vi "GraphViz Generator UI Wrapper.vi"(10 "Modules Configurations":refnum<class "TBM module configuration.lvclass">[](array[class]), 11 "engine configuration in":refnum<class "engine configuration.lvclass">) -> ()   [LabVIEW 2013, in "GraphViz Mapping Visualizer.lvlib"]
uses:
  GraphViz Mapping Visualizer.lvlib
  <vilib>/NI/Module Execution Interface/Engine Configuration/engine configuration.lvclass
  <vilib>/NI/Tag Bus Module Framework/module configuration/TBM module configuration.lvclass
  System.Windows.Forms
  <vilib>/event_ctls.llb/panelstate.ctl
  <vilib>/event_ctls.llb/sizeaction.ctl
  System.Drawing
  Configuration Editor/Classes/Engine Mappings/Engine Mappings.lvclass
panel:
  in  "Tab Control":enum32{"Setup", "Image"}(tab)
  in  "Modules to View":T1(array[cluster])
  in  "Supported Colors":string[](array[string])=["dodgerblue", "cadetblue1", "darkgoldenrod1", "gainsboro", "palegreen", "peachpuff", "violet", "skyblue", "yellow", "seagreen1", "tomato", "thistle", "slateblue1", "orange", "palevioletred1"]
  in  "Show Unmapped Channels?":bool=TRUE
  in  "Show Tag Labels?":bool
  in  "Zoom?":bool=TRUE
  in  "Generate":bool
  in  "PictureBox":refnum<k24>(container)
  # "Generation Options"
  # "Supported colors list found at \nhttp://www.graphviz.org/doc/info/colors.html"
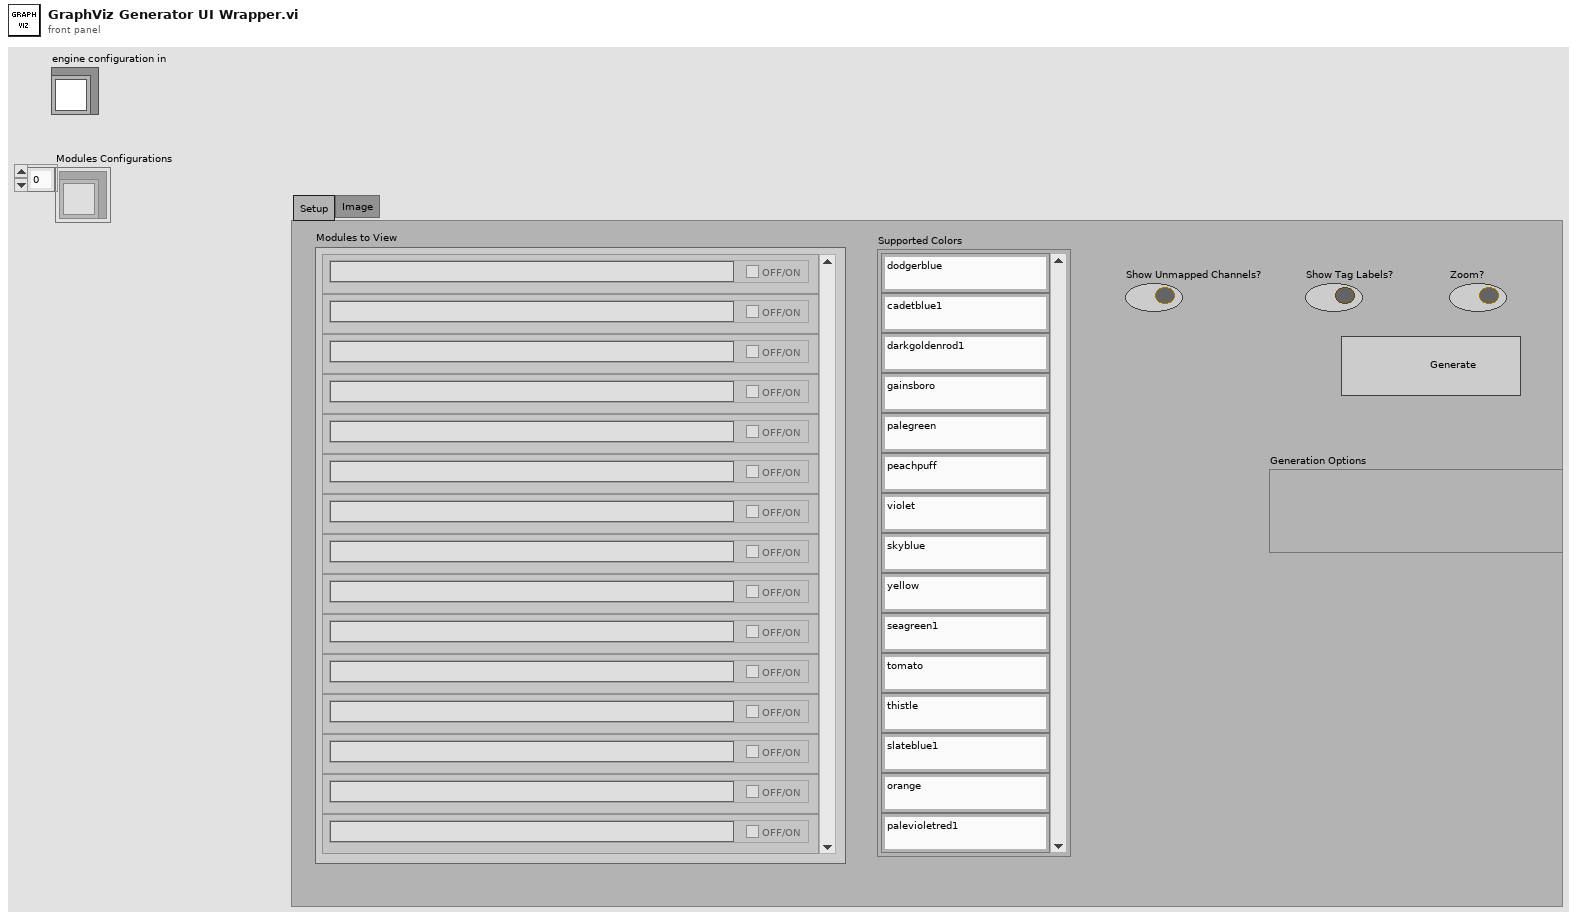
[diagram p1: front panel]
types:
  T1 = cluster{"Module Display Name":string, "View?":bool}[]
  T2 = typedef "PL Framework Configuration Tool.lvlib/Engine Mappings.lvclass/module information.ctl" = cluster{"display name":string, "instance id":string, "channels":refnum<class "TBM channel.lvclass">[]}
  T3 = cluster{"Module Display Name":string, "View?":bool}
  T4 = enum16{"open", "replace", "create", "open or create", "replace or create", "replace or create with confirmation"}
  T5 = typedef "sizeaction.ctl" = enum32{"Minimized", "Maximized", "Resized"}
  T6 = typedef "panelstate.ctl" = enum32{"Standard", "Minimized", "Maximized"}
  T7 = typedef "LVRectTypeDef.ctl" = cluster{"Left":i16, "Top":i16, "Right":i16, "Bottom":i16}
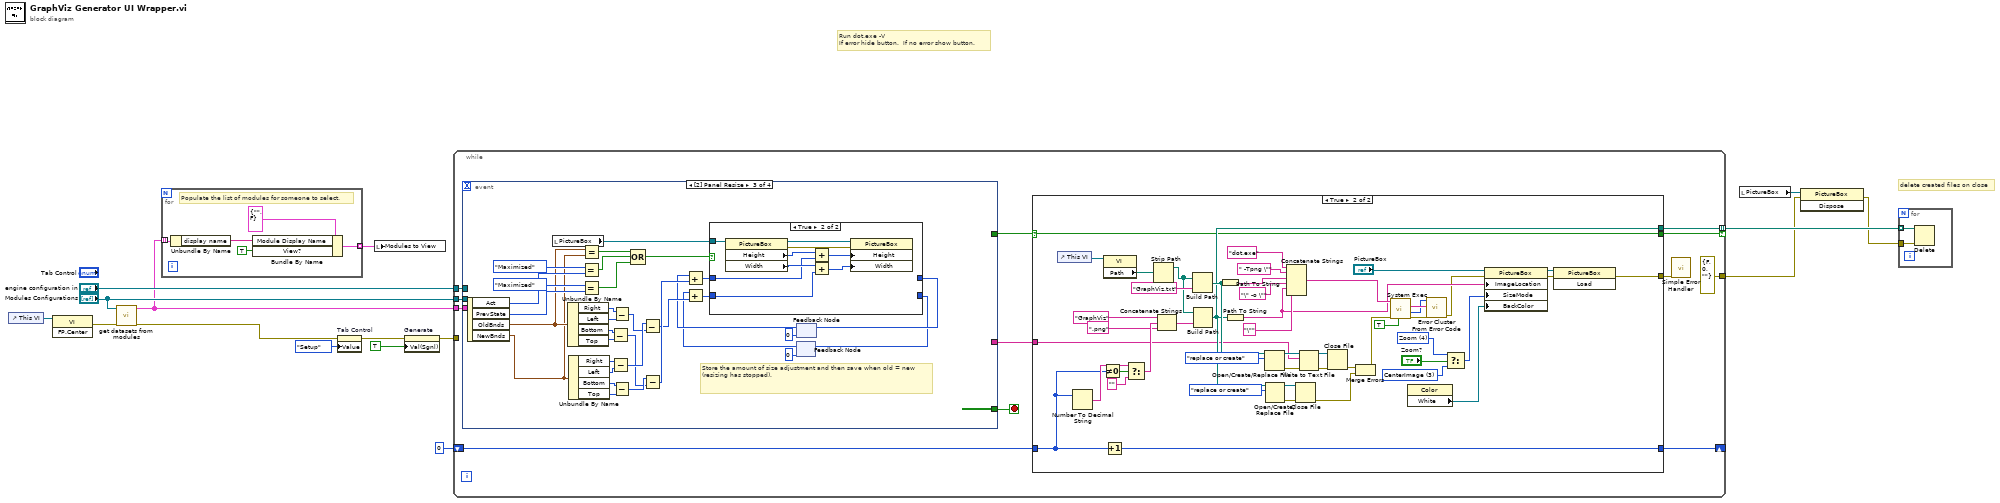
[diagram p0: block diagram]
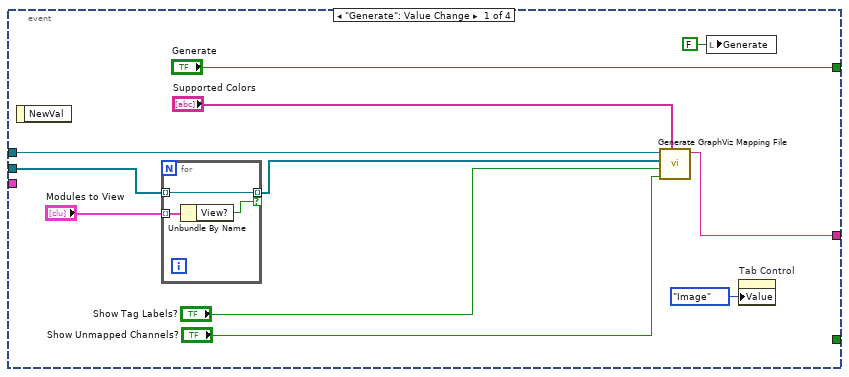
[diagram p3: hidden frame]
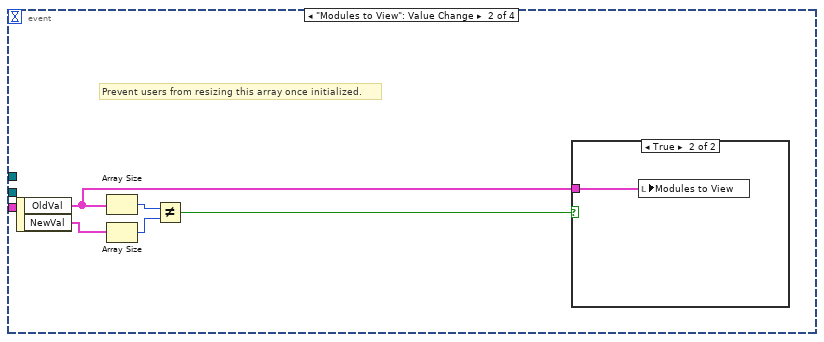
[diagram p4: hidden frame]
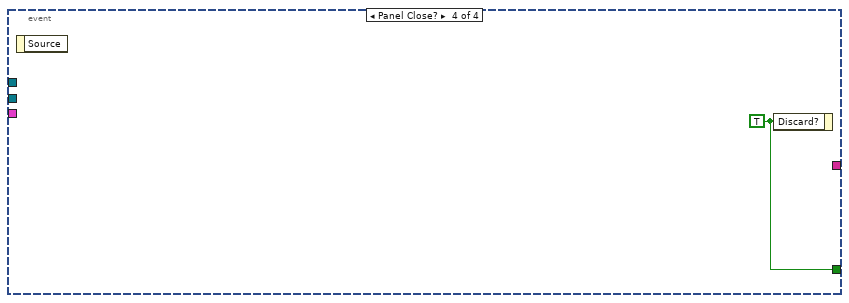
[diagram p7: hidden frame]
diagram:
  # "Run dot.exe -V\nIf error hide button.  If no error show button."
  # "delete created files on close"
  n1 = control-ref of="This VI"() -> (w2:refnum<vi>)
  n2 = invoke class="VI" method="FP.Center"(reference=w2) -> (error out=w1:errorcluster)  [unwired: 2 in, 2 out]
  n3 = call "get datasets from modules.vi"("error in"=w1, "Modules Configurations"="Modules Configurations") -> ("error out"=w4:errorcluster, "module datasets"=w12:T2[])  [unwired: 8 in]
  n4 = for {
    tunnel: w12 -> [w21] mode=indexing
    tunnel: [w17] -> w11 mode=indexing
    # "Populate the list of modules for someone to select."
    n5 = Unbundle By Name(w21) -> ("display name"=w18:string)
    n6 = Bundle By Name(cluster=T3 {"Module Display Name"="", "View?"=FALSE} ("Cluster"), "Module Display Name"=w18, "View?"=TRUE) -> (w17:T3)
  }
  n7 = property on="Tab Control" class="TabCtl (strict)"(error in=w4, "Value"=enum32{"Setup", "Image", "Text"}."Setup" ("Tab Control")) -> (error out=w6:errorcluster)  [unwired: 1 in, 1 out]
  n8 = local write "Modules to View"(w11) -> ()
  n9 = property on="Generate" class="Bool (strict)"(error in=w6, "Val(Sgnl)"=TRUE) -> (error out=w3:errorcluster)  [unwired: 1 in, 1 out]
  n10 = while {
    tunnel: "engine configuration in" -> [w33]
    tunnel: "Modules Configurations" -> [w32]
    shift-right: [w28] -> _
    shift-left: 0 -> [w27]
    tunnel: [w26] -> w14 mode=indexing if=w25
    tunnel: w12 -> [w24]
    tunnel: [errorcluster {"status"=FALSE, "code"=0, "source"=""} ("error out")] -> w9
    tunnel: w3 -> [_]
    stop <- w31 stop-if-true
    n11 = event shown="[2] Panel Resize" {
      selector: _ -> [_ _ _ _]
      dyn-events: _ -> [_ _ _ _]
      timeout: _ -> [_ _ _ _]
      tunnel: w33 -> [w89 _ _ _]
      tunnel: w32 -> [w88 _ _ _]
      tunnel: [_ _ _ w148] -> w31
      tunnel: ["Generate" _ _ _] -> w30
      tunnel: [w90 _ _ _] -> w29
      tunnel: w24 -> [_ _ _ _]
      event "Generate": Value Change {
        n12 = event-data() -> ()  [unwired: 1 in, 1 out]
        n13 = for {
          tunnel: "Modules to View" -> [w97] mode=indexing
          tunnel: w88 -> [w96] mode=indexing
          tunnel: [w96] -> w87 mode=indexing if=w95
          n14 = Unbundle By Name(w97) -> ("View?"=w95:bool)
        }
        n15 = call "Generate GraphViz Mapping File.vi"("supported colors"="Supported Colors", "Show Unmapped Channels?"="Show Unmapped Channels?", "Show Tag Labels?"="Show Tag Labels?", "Modules Configurations"=w87, "engine configuration in"=w89) -> ("output to graphviz"=w90:string)  [unwired: 6 in]
        n16 = local write "Generate"(FALSE ("Generate")) -> ()
        n17 = property on="Tab Control" class="TabCtl (strict)"("Value"=enum32{"Setup", "Image", "Text"}."Image" ("Tab Control")) -> ()  [unwired: 2 in, 2 out]
      }
      event "Modules to View": Value Change {
        # "Prevent users from resizing this array once initialized."
        n18 = event-data() -> ("OldVal"=w98:T1, "NewVal"=w102:T1)  [unwired: 1 in]
        n19 = Array Size(array=w98) -> (size(s)=w101:i32)
        n20 = Array Size(array=w102) -> (size(s)=w100:i32)
        n21 = Not Equal?(x=w101, y=w100) -> (x != y?=w99:bool)
        n22 = case shown="True" w99 {
          tunnel: w98 -> [_ w103]
          frame False {
          }
          frame True {
            n23 = local write "Modules to View"(w103) -> ()
          }
        }
      }
      event Panel Resize {
        # "Store the amount of size adjustment and then save when old = new (resizing has stopped)."
        n24 = event-data() -> ("Act"=w108:T5, "PrevState"=w107:T6, "OldBnds"=w106:T7, "NewBnds"=w105:T7)  [unwired: 1 in]
        n25 = local read "PictureBox"() -> (w104:refnum<k24>)
        n26 = Unbundle By Name(w106) -> ("Right"=w119:i16, "Left"=w120:i16, "Bottom"=w118:i16, "Top"=w117:i16)
        n27 = Unbundle By Name(w105) -> ("Right"=w116:i16, "Left"=w115:i16, "Bottom"=w114:i16, "Top"=w113:i16)
        n28 = Equal?(x=sizeaction."Maximized" ("Act"), y=w108) -> (x = y?=w124:bool)
        n29 = Equal?(x=panelstate."Maximized", y=w107) -> (x = y?=w123:bool)
        n30 = Equal?(x=w106, y=w105) -> (x = y?=w125:bool)
        n31 = Subtract(x=w118, y=w117) -> (x-y=w109:i16)
        n32 = Subtract(x=w116, y=w115) -> (x-y=w112:i16)
        n33 = Subtract(x=w119, y=w120) -> (x-y=w111:i16)
        n34 = Subtract(x=w114, y=w113) -> (x-y=w110:i16)
        n35 = Compound Arithmetic op=OR(w125, w124, w123) -> (w122:bool)
        n36 = Subtract(x=w112, y=w111) -> (x-y=w135:i16)
        n37 = Subtract(x=w110, y=w109) -> (x-y=w136:i16)
        n38 = feedback #1(0 ("x+y")) -> (w129:i32)
        n39 = Add(x=w129, y=w135) -> (x+y=w131:i32)
        n40 = feedback #2(0 ("x+y")) -> (w130:i32)
        n41 = Add(x=w130, y=w136) -> (x+y=w132:i32)
        n42 = case shown="True" w122 {
          tunnel: w104 -> [_ w141]
          tunnel: w132 -> [w138 w140]
          tunnel: w131 -> [w137 w139]
          tunnel: [w138 _] -> w128
          tunnel: [w137 _] -> w127
          frame False {
          }
          frame True {
            n43 = property class="PictureBox"(reference=w141) -> (reference out=w147:refnum<k24>, error out=w142:errorcluster, "Height"=w146:i32, "Width"=w145:i32)  [unwired: 1 in]
            n44 = Add(x=w146, y=w140) -> (x+y=w144:i32)
            n45 = Add(x=w145, y=w139) -> (x+y=w143:i32)
            n46 = property class="PictureBox"(reference=w147, error in=w142, "Height"=w144, "Width"=w143) -> ()  [unwired: 2 out]
          }
        }
        n47 = feedback-in #1(w127) -> ()
        n48 = feedback-in #2(w128) -> ()
      }
      event Panel Close? {
        w148 = TRUE ("Discard?")
        n49 = event-data() -> ()  [unwired: 1 in, 1 out]
        n50 = event-data("Discard?"=w148) -> ()  [unwired: 1 in, 1 out]
      }
    }
    n51 = case shown="True" w30 {
      selector: w30 -> [_ w43]
      tunnel: w29 -> [_ w36]
      tunnel: w27 -> [w34 w51]
      tunnel: [w34 w50] -> w28
      tunnel: [_ w44] -> w26
      tunnel: [_ w43] -> w25
      tunnel: [_ w41] -> w23
      frame False {
      }
      frame True {
        w48 = 4 items=["Normal", "StretchImage", "AutoSize", "CenterImage", "Zoom"] ("SizeMode")
        w47 = 3 items=["Normal", "StretchImage", "AutoSize", "CenterImage", "Zoom"] ("SizeMode")
        n52 = control-ref of="This VI"() -> (w77:refnum<vi>)
        n53 = Number To Decimal String(number=w51) -> (decimal integer string=w58:string)  [unwired: 1 in]
        n54 = Not Equal To 0?(x=w51) -> (x != 0?=w59:bool)
        n55 = property class="VI"(reference=w77) -> ("Path"=w78:path)  [unwired: 1 in, 2 out]
        n56 = Increment(x=w51) -> (x+1=w50:i32)
        n57 = Select(t=w58, s=w59, f="") -> (s? t:f=w55:string)
        n58 = Strip Path(path=w78) -> (stripped path=w45:path)  [unwired: 1 out]
        n59 = Concatenate Strings("GraphViz" ("name or relative path"), w55, ".png" ("string")) -> (w53:string)
        n60 = Build Path(base path=w45, name or relative path="GraphViz.txt") -> (appended path=w66:path)
        n61 = Build Path(base path=w45, name or relative path=w53) -> (appended path=w44:path)
        n62 = Path To String(path=w66) -> (string=w80:string)
        n63 = Path To String(path=w44) -> (string=w61:string)
        n64 = Open/Create/Replace File(file path (use dialog)=w66, operation (0:open)=T4."replace or create") -> (refnum out=w72:refnum<file>, error out=w71:errorcluster)  [unwired: 4 in, 1 out]
        n65 = Open/Create/Replace File(file path (use dialog)=w44, operation (0:open)=T4."replace or create") -> (refnum out=w73:refnum<file>, error out=w74:errorcluster)  [unwired: 4 in, 1 out]
        n66 = Concatenate Strings("dot.exe" ("name or relative path"), " -Tpng \"" ("string"), w80, "\" -o \"" ("string"), w61, "\"" ("string")) -> (w65:string)
        n67 = Close File(refnum=w73, error in=w74) -> (error out=w67:errorcluster)  [unwired: 1 out]
        n68 = Write to Text File(file (use dialog)=w72, text=w36, error in=w71) -> (refnum out=w69:refnum<file>, error out=w70:errorcluster)  [unwired: 1 in, 1 out]
        n69 = Close File(refnum=w69, error in=w70) -> (error out=w68:errorcluster)  [unwired: 1 out]
        n70 = Merge Errors(w68, w67) -> (w64:errorcluster)
        n71 = call <vilib>:"System Exec.vi"("run minimized? (F)"=TRUE, "error in (no error)"=w64, "command line"=w65) -> ("error out"=w40:errorcluster, "return code"=w38:i32, "standard error"=w39:string)  [unwired: 5 in, 1 out]
        n72 = property class="Color"() -> ("White"=w52:refnum<k24>)  [unwired: 2 in, 2 out]
        n73 = call <vilib>:"Error Cluster From Error Code.vi"("error in (no error)"=w40, "error message (\"\")"=w39, "error code (0)"=w38) -> ("error out"=w37:errorcluster)  [unwired: 6 in]
        n74 = Select(t=w48, s="Zoom?", f=w47) -> (s? t:f=w46:i32)
        n75 = property class="PictureBox"(reference="PictureBox", error in=w37, "ImageLocation"=w61, "SizeMode"=w46, "BackColor"=w52) -> (reference out=w62:refnum<k24>, error out=w60:errorcluster)
        n76 = invoke class="PictureBox" method="Load"(reference=w62, error in=w60) -> (error out=w41:errorcluster)  [unwired: 1 in, 2 out]
      }
    }
    n77 = call <vilib>:"Simple Error Handler.vi"("error in (no error)"=w23) -> ()  [unwired: 4 in, 5 out]
  }
  n78 = local read "PictureBox"() -> (w10:refnum<k24>)
  n79 = invoke class="PictureBox" method="Dispose"(reference=w10, error in=w9) -> (error out=w8:errorcluster)  [unwired: 1 in, 2 out]
  n80 = for {
    tunnel: w14 -> [w150] mode=indexing
    tunnel: w8 -> [w149]
    n81 = Delete(path (use dialog)=w150, error in=w149) -> ()  [unwired: 3 in, 3 out]
  }
